vi "RTS Runtime Save.vi"(4 "File Size":dbl=15.0 format="%#_13g", 6 "Custom Saved Titles":string[][](array[string]), 8 "error in (no error)":errorcluster, 9 "Setup Info Station 8":string[][](array[string]), 10 "CSV File Location Input":path, 11 "Byte Stream File in":refnum<file>) -> (0 "error out":errorcluster, 2 "CSV File Location Output":path, 3 "Byte Stream File out":refnum<file>)   [LabVIEW 2016]
uses:
  Utility/Save File/Save File.lvlib
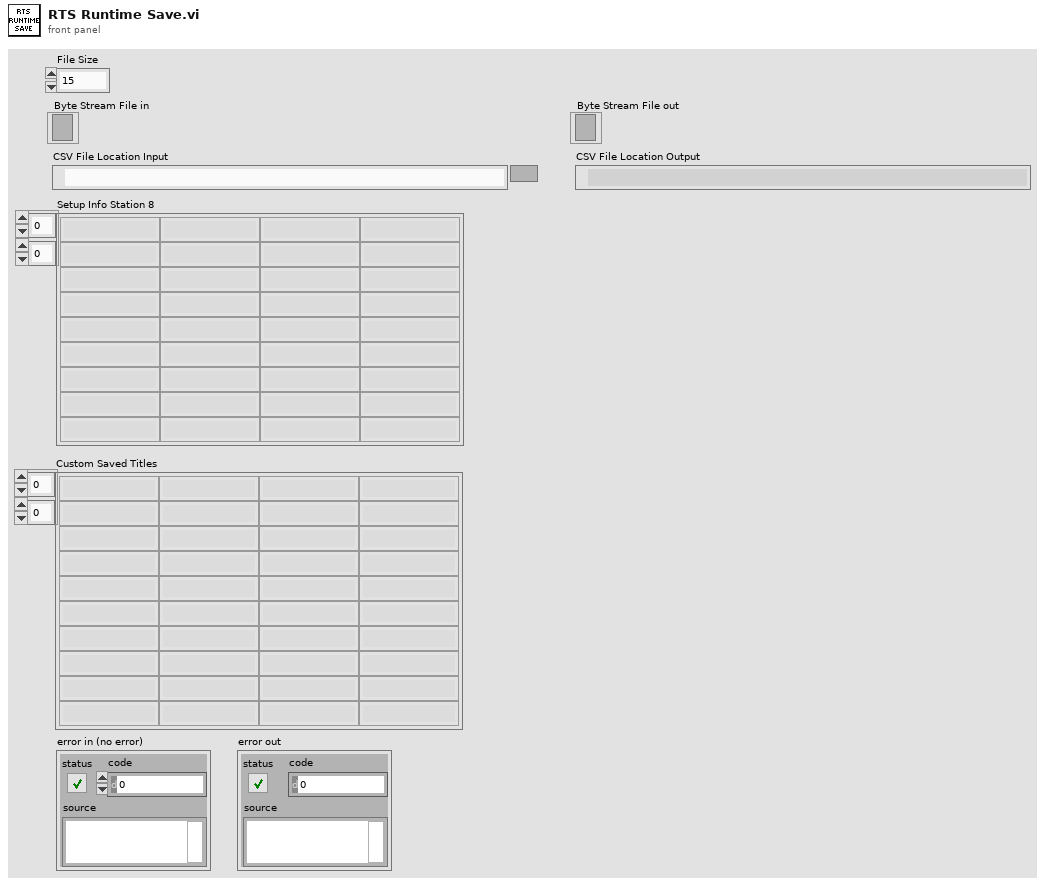
[diagram p1: front panel]
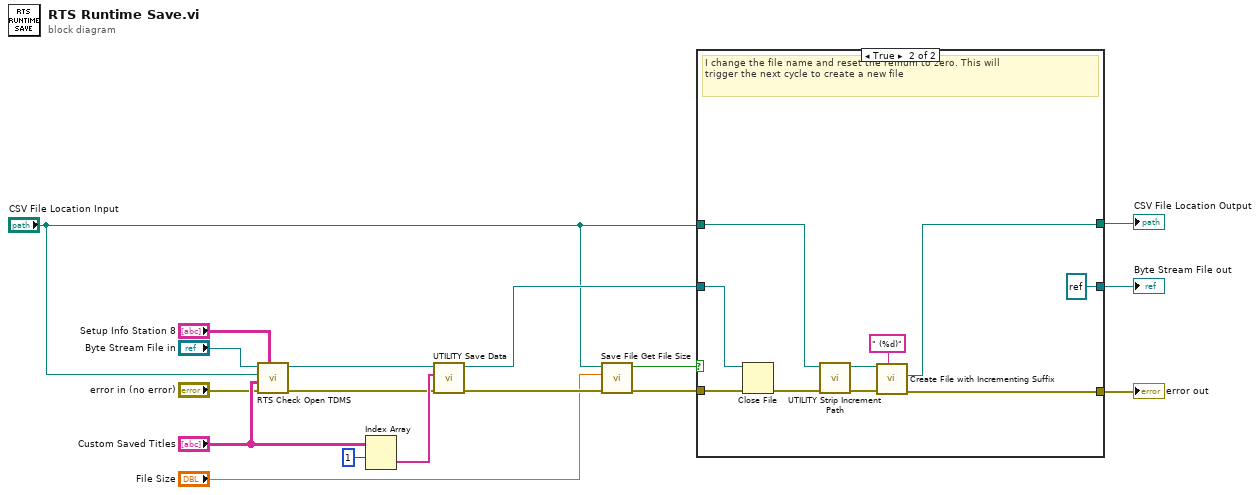
[diagram p0: block diagram]
diagram:
  n1 = call "RTS Check Open TDMS.vi"("Setup Info Station #"="Setup Info Station 8", "error in (no error)"="error in (no error)", "Data"="Custom Saved Titles", "CSV File Location"="CSV File Location Input", "Byte Stream File In"="Byte Stream File in") -> ("error out"=w10:errorcluster, "Byte Stream File Out"=w14:refnum<file>)  [unwired: 4 in, 1 out]
  n2 = Index Array(array="Custom Saved Titles", index (row)=1) -> (element=w12:string[])  [unwired: 1 in]
  n3 = call "UTILITY Save Data.vi"("error in"=w10, "Data"=w12, "refnum"=w14) -> ("error out"=w17:errorcluster, "refnum out"=w6:refnum<file>)  [unwired: 7 in]
  n4 = call "Save File Get File Size.vi"("Error In"=w17, "File Size"="File Size", "Old path"="CSV File Location Input") -> ("Error Out"=w5:errorcluster, "File Size Greater Than Limit"=w7:bool)  [unwired: 6 in, 1 out]
  n5 = case shown="True" w7 {
    tunnel: w6 -> [w20 w30]
    tunnel: w5 -> [w19 w29]
    tunnel: "CSV File Location Input" -> [w18 w24]
    tunnel: [w18 w28] -> w1
    tunnel: [w19 w27] -> w3
    tunnel: [w20 refnum<file> refnum ("refnum out")] -> w2
    frame False {
    }
    frame True {
      # "I change the file name and reset the refnum to zero. This will\ntrigger the next cycle to create a new file"
      n6 = Close File(refnum=w30, error in=w29) -> (error out=w22:errorcluster)  [unwired: 1 out]
      n7 = call "UTILITY Strip Increment Path.vi"("Error In"=w22, "file path in"=w24) -> ("Error Out"=w21:errorcluster, "file path out"=w23:path)  [unwired: 8 in]
      n8 = call <vilib>:"Create File with Incrementing Suffix.vi"("format string (\" (%d)\")"=" (%d)" ("format string (\" (%d)\")"), "error in (no error)"=w21, "file path"=w23) -> ("error out"=w27:errorcluster, "actual path"=w28:path)  [unwired: 6 in, 1 out]
    }
  }
  "error out" <- w3
  "Byte Stream File out" <- w2
  "CSV File Location Output" <- w1
